vi "Enter ROI Name.vi"() -> ()   [LabVIEW 2014, in "POLARIS IMAQ Display.xctl"]
uses:
  POLARIS IMAQ Display.xctl
panel:
  in  "ref":refnum<vi>
  in  "Enter ROI Name":string
  in  "Stop":bool
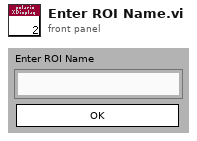
[diagram p1: front panel]
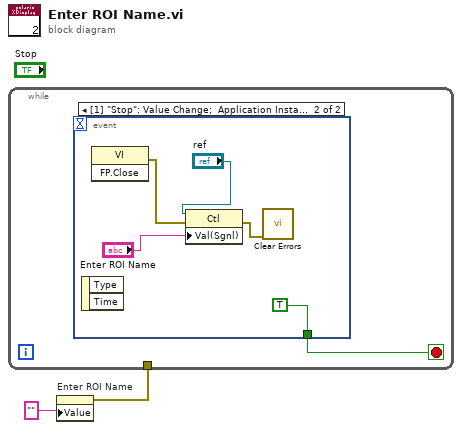
[diagram p0: block diagram]
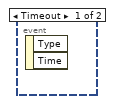
[diagram p2: hidden frame]
diagram:
  n1 = property on="Enter ROI Name" class="Str"("Value"="" ("Enter ROI Name")) -> (error out=w1:errorcluster)  [unwired: 2 in, 1 out]
  n2 = while {
    tunnel: w1 -> [_]
    stop <- w3 stop-if-true
    n3 = event shown="[1] \"Stop\": Value Change;  Application Instance Close" {
      selector: _ -> [_ _]
      dyn-events: _ -> [_ _]
      timeout: _ -> [_ _]
      tunnel: [_ TRUE] -> w3
      event Timeout {
        n4 = event-data() -> ()  [unwired: 1 in, 2 out]
      }
      event "Stop": Value Change; Application Instance Close {
        n5 = event-data() -> ()  [unwired: 1 in, 2 out]
        n6 = invoke class="VI" method="FP.Close"() -> (error out=w5:errorcluster)  [unwired: 3 in, 2 out]
        n7 = property class="Ctl"(reference="ref", error in=w5, "Val(Sgnl)"="Enter ROI Name") -> (error out=w6:errorcluster)  [unwired: 1 out]
        n8 = call <vilib>:"Clear Errors.vi"("error in (no error)"=w6) -> ()  [unwired: 5 in, 2 out]
      }
    }
  }
